vi "Email küldése  - Szöveges + Csatolmány.vi"() -> ()   [LabVIEW 2020]
uses:
  <vilib>/smtpClient/Set Message Text.vi
  <vilib>/smtpClient/LabVIEWSMTPClient.lvlib
panel:
  in  "Üzenet":string
  in  "Tárgy":string
  in  "Kinek küldöd az emailt:":string
  in  "attachments":path[](array[path])
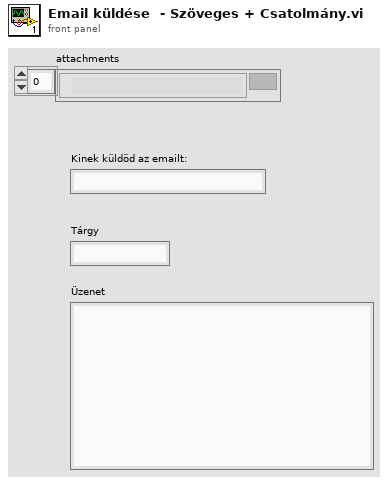
[diagram p1: front panel]
types:
  T1 = typedef "LabVIEWSMTPClient.lvlib/SmtpClientHandle.ctl" = refnum<k1>
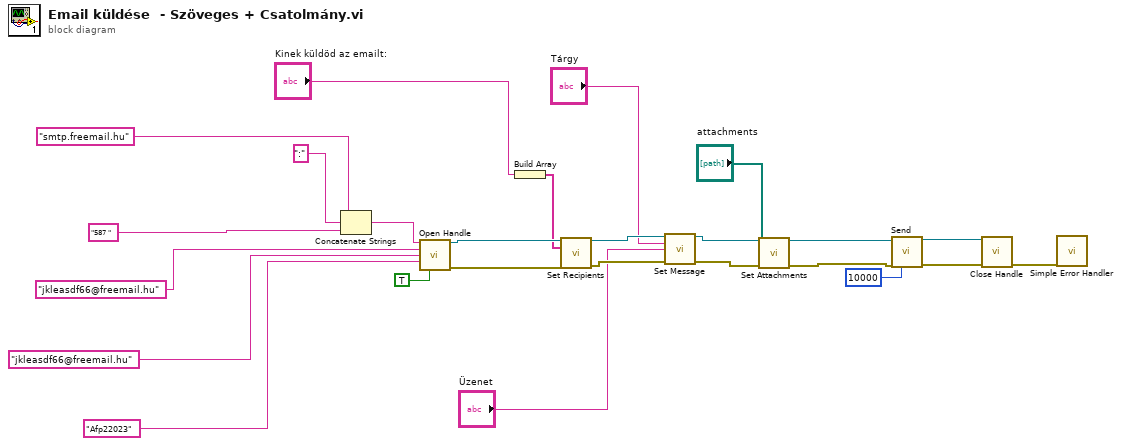
[diagram p0: block diagram]
diagram:
  n1 = Concatenate Strings("smtp.freemail.hu" ("string"), ":" ("string"), "587 " ("string")) -> (w22:string)
  n2 = call <vilib>:"Open Handle.vi"("server address"=w22, "from"="jkleasdf66@freemail.hu" ("username"), "username"="jkleasdf66@freemail.hu", "password"="Afp22023", "use TLS (false)"=TRUE) -> ("handle out"=w25:T1, "error out"=w12:errorcluster)  [unwired: 9 in]
  n3 = Build Array("Kinek küldöd az emailt:") -> (w4:string[])
  n4 = call <vilib>:"Set Recipients.vi"("handle in"=w25, "to"=w4, "error in (no error)"=w12) -> ("handle out"=w24:T1, "error out"=w11:errorcluster)  [unwired: 11 in]
  n5 = call-poly <vilib>:"Set Message.vi"("handle in"=w24, "subject"="Tárgy", "plain text message"="Üzenet", "error in (no error)"=w11) -> ("handle out"=w14:T1, "error out"=w10:errorcluster)  [unwired: 10 in]
  n6 = call <vilib>:"Set Attachments.vi"("handle in"=w14, "attachments"="attachments", "error in (no error)"=w10) -> ("handle out"=w13:T1, "error out"=w9:errorcluster)  [unwired: 11 in]
  n7 = call <vilib>:"Send.vi"("handle in"=w13, "error in (no error)"=w9, "timeout in ms (10000)"=10000) -> ("handle out"=w23:T1, "error out"=w8:errorcluster)  [unwired: 10 in, 1 out]
  n8 = call <vilib>:"Close Handle.vi"("handle in"=w23, "error in (no error)"=w8) -> ("error out"=w6:errorcluster)  [unwired: 12 in, 1 out]
  n9 = call <vilib>:"Simple Error Handler.vi"("error in (no error)"=w6) -> ()  [unwired: 4 in, 5 out]
